vi "ics_save_3D.vi"(0 "pixels":i32, 1 "filename":string, 3 "folder":path=path "D:/User/Sergey/ids_ics_trainer", 5 "Dwell":dbl, 7 "slices Z":i32, 9 "Range Z":dbl, 11 "Range":dbl, 12 "scale I":i32=1) -> (4 "saved":bool, 6 "path to .ids":path, 15 "error out":errorcluster)   [LabVIEW 2009]
panel:
  in  "error in":errorcluster
  out "text":string
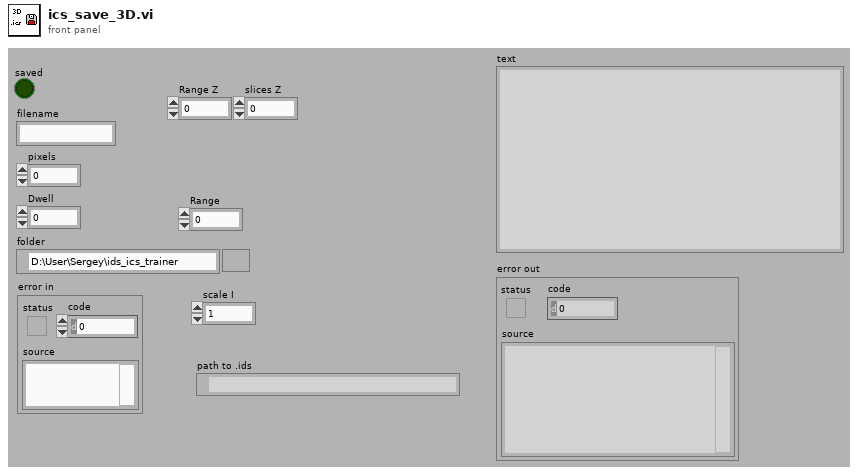
[diagram p1: front panel]
types:
  T1 = enum16{"open", "replace", "create", "open or create", "replace or create", "replace or create with confirmation"}
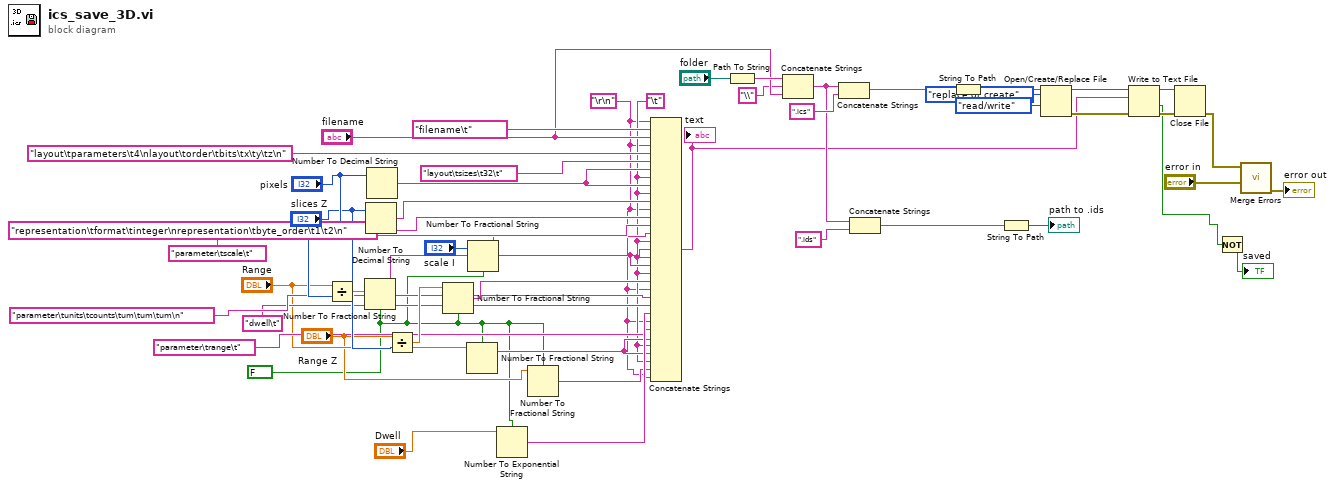
[diagram p0: block diagram]
diagram:
  w7 = FALSE ("use system decimal point (T)")
  w6 = "\t"
  w4 = "\r\n"
  n1 = Divide(x="Range", y="pixels") -> (x/y=w24:dbl)
  n2 = Number To Fractional String(use system decimal point (T)=w7, number=w24) -> (F-format string=w21:string)  [unwired: 2 in]
  n3 = Number To Decimal String(number="slices Z") -> (decimal integer string=w28:string)  [unwired: 1 in]
  n4 = Number To Decimal String(number="pixels") -> (decimal integer string=w29:string)  [unwired: 1 in]
  n5 = Divide(x="Range Z", y="slices Z") -> (x/y=w19:dbl)
  n6 = Number To Fractional String(use system decimal point (T)=w7, number=w19) -> (F-format string=w18:string)  [unwired: 2 in]
  n7 = Number To Fractional String(use system decimal point (T)=w7, number="Range") -> (F-format string=w11:string)  [unwired: 2 in]
  n8 = Number To Fractional String(use system decimal point (T)=w7, number="scale I") -> (F-format string=w22:string)  [unwired: 2 in]
  n9 = Number To Exponential String(number="Dwell", 1:w7) -> (E-format string=w14:string)  [unwired: 2 in]
  n10 = Number To Fractional String(use system decimal point (T)=w7, number="Range Z") -> (F-format string=w5:string)  [unwired: 2 in]
  n11 = Concatenate Strings(w4, "filename\t" ("string"), "filename", w4, "layout\tparameters\t4\nlayout\torder\tbits\tx\ty\tz\n" ("string"), "layout\tsizes\t32\t" ("string"), w29, w6, w29, w6, w28, w4, "representation\tformat\tinteger\nrepresentation\tbyte_order\t1\t2\n" ("string"), "parameter\tscale\t" ("string"), w22, w6, w21, w6, w21, w6, w18, w4, "parameter\tunits\tcounts\tum\tum\tum\n" ("string"), "dwell\t" ("string"), w14, w4, "parameter\trange\t" ("string"), w11, w6, w11, w6, w5, w4) -> (w34:string)
  "text" <- w34
  n12 = Path To String(path="folder") -> (string=w43:string)
  n13 = Concatenate Strings(w43, "\\" ("string"), "filename") -> (w36:string)
  n14 = Concatenate Strings(w36, ".ics" ("string")) -> (w38:string)
  n15 = Concatenate Strings(w36, ".ids" ("string")) -> (w35:string)
  n16 = String To Path(string=w38) -> (path=w42:path)
  n17 = String To Path(string=w35) -> (path=→"path to .ids":path)
  n18 = Open/Create/Replace File(file path (use dialog)=w42, operation (0:open)=T1."replace or create", access (0:read/write)=enum16{"read/write", "read-only", "write-only"}."read/write") -> (refnum out=w45:refnum<file>, error out=w44:errorcluster)  [unwired: 3 in, 1 out]
  n19 = Write to Text File(file (use dialog)=w45, text=w34, error in=w44) -> (refnum out=w47:refnum<file>, cancelled=w3:bool, error out=w46:errorcluster)  [unwired: 1 in]
  n20 = Close File(refnum=w47, error in=w46) -> (error out=w33:errorcluster)  [unwired: 1 out]
  n21 = Not(x=w3) -> (.not. x?=→"saved":bool)
  n22 = call <vilib>:"Merge Errors.vi"("error in 3 (no error)"="error in", "error in 1 (no error)"=w33) -> ("error out"=→"error out":errorcluster)  [unwired: 5 in]
